vi "Memory.Pointer.New Subset Pointer.vi"(8 "error in (no error)":errorcluster, 9 "length":u64 format="%d bytes", 10 "offset":u64 format="%d bytes", 11 "Pointer in":refnum<class "Memory.Pointer.Void.lvclass">) -> (0 "error out":errorcluster, 2 "subset Pointer":refnum<class "Memory.Pointer.Void.lvclass">, 3 "Pointer out":refnum<class "Memory.Pointer.Void.lvclass">)   [LabVIEW 2016, in "LabVIEW Memory Manager.lvlib" / "Memory.Pointer.Void.lvclass"]
uses:
  Memory.Pointer.Void.lvclass
  Memory.Pointer.Void.lvclass/Memory.Pointer.Void.ctl
  Memory.Pointer.Set Address.vi
  Memory.Pointer.Offset to Address.Safe.vi
  Memory.Pointer.Get Size.vi
  Memory.Pointer.Parameter Check.Length.vi
  Memory.Pointer.Parameter Check.Offset.vi
  Memory.Pointer.Offset to Address.Unsafe.vi
  Memory.Pointer.Get Address.vi
  Memory.Pointer.Error Handling.Out of Range.vi
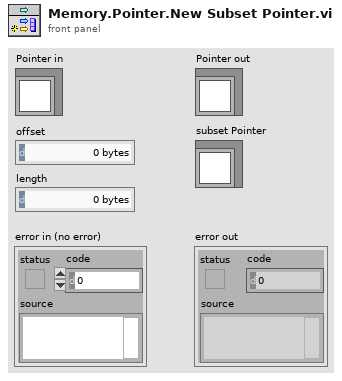
[diagram p1: front panel]
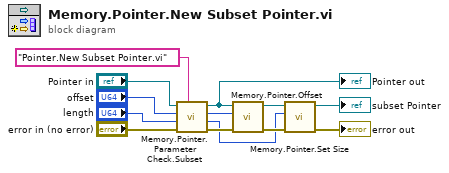
[diagram p0: block diagram]
diagram:
  n1 = call "Memory.Pointer.Parameter Check.Subset.vi"("calling vi name"="Pointer.New Subset Pointer.vi", "error in (no error)"="error in (no error)", "length"="length", "offset"="offset", "Pointer in"="Pointer in") -> ("error out"=w13:errorcluster, "length out"=w2:u64, "offset out"=w7:u64, "Pointer out"=w8:refnum<class "Memory.Pointer.Void.lvclass">)  [unwired: 3 in]
  "Pointer out" <- w8
  n2 = call "Memory.Pointer.Offset.vi"("error in (no error)"=w13, "offset"=w7, "Pointer in"=w8) -> ("error out"=w5:errorcluster, "Pointer out"=w6:refnum<class "Memory.Pointer.Void.lvclass">)  [unwired: 7 in]
  n3 = call "Memory.Pointer.Set Size.vi"("error in (no error)"=w5, "size"=w2, "Pointer in"=w6) -> ("error out"=→"error out":errorcluster, "Pointer out"=→"subset Pointer":refnum<class "Memory.Pointer.Void.lvclass">)  [unwired: 7 in]
